vi "Generate User Event.vi"(6 "Add(t)/Remove(f) Event":bool, 8 "error in (no error)":errorcluster, 9 "User Event in":refnum<user-event>, 10 "Status Array In":string[](array[string]), 11 "Error Codes":T1) -> (0 "error out":errorcluster, 3 "User Event out":refnum<user-event>)   [LabVIEW 2011]
uses:
  User Event Data Type typdef.ctl
  Error Action.ctl
  Error codes.ctl
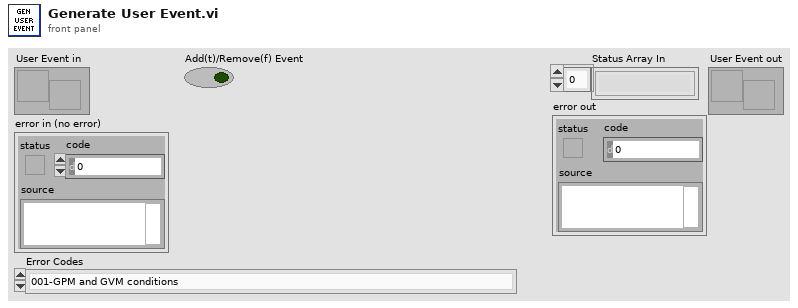
[diagram p1: front panel]
types:
  T1 = typedef "Error codes.ctl" = enum16{"001-GPM and GVM conditions", "002-Turbo gate valve status", "003-Chamber Gate Valve Status", "004-Check Chamber Pressures", "005-Check GPM Handshake", "006-Roughing Pump Status", "007-Backing Pump Status", "008-Backing valve status", "009-Roughing Manifold Pressure Status", "010-Roughing Valve Status", "011-Roughing Pump Status", "012-Turbo Backing Valve Status", "013-MID-VAC Status", "999-No Event"}
  T2 = typedef "User Event Data Type typdef.ctl" = cluster{"Error Action":T3, "Error Codes":T1, "Status Array":string[]}
  T3 = typedef "Error Action.ctl" = enum16{"Add", "Remove", "Read All"}
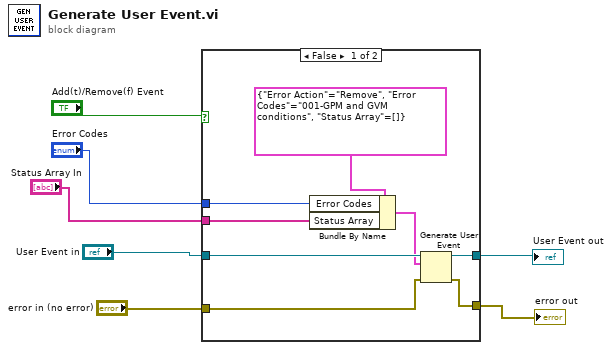
[diagram p0: block diagram]
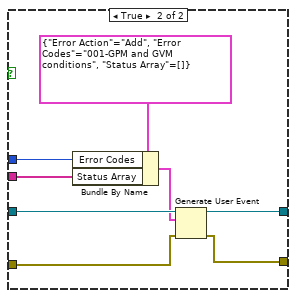
[diagram p2: hidden frame]
diagram:
  n1 = case shown="False" "Add(t)/Remove(f) Event" {
    tunnel: "User Event in" -> [w14 w23]
    tunnel: "error in (no error)" -> [w13 w22]
    tunnel: [w12 w21] -> w1
    tunnel: [w15 w20] -> w2
    tunnel: "Error Codes" -> [w10 w17]
    tunnel: "Status Array In" -> [w8 w16]
    frame False {
      n2 = Bundle By Name(cluster=T2 {"Error Action"=enum."Remove", "Error Codes"=enum."001-GPM and GVM conditions", "Status Array"=[]} ("User Event data type"), "Error Codes"=w10, "Status Array"=w8) -> (w9:T2)
      n3 = Generate User Event(user event=w14, event data cluster=w9, error in=w13) -> (user event out=w15:refnum<user-event>, error out=w12:errorcluster)
    }
    frame True {
      n4 = Bundle By Name(cluster=T2 {"Error Action"=enum."Add", "Error Codes"=enum."001-GPM and GVM conditions", "Status Array"=[]} ("User Event data type"), "Error Codes"=w17, "Status Array"=w16) -> (w18:T2)
      n5 = Generate User Event(user event=w23, event data cluster=w18, error in=w22) -> (user event out=w20:refnum<user-event>, error out=w21:errorcluster)
    }
  }
  "error out" <- w1
  "User Event out" <- w2
